vi "HW_GEN - Write Module Channel Configurations(bin).vi"(8 "error in":errorcluster caption="错误输入", 10 "ModuCfg":T1[](array[typedef]), 11 "Path":path) -> (0 "error out":errorcluster caption="错误输出")   [LabVIEW 2016]
uses:
  Ctrls/HardWare _ Module Configuration.ctl
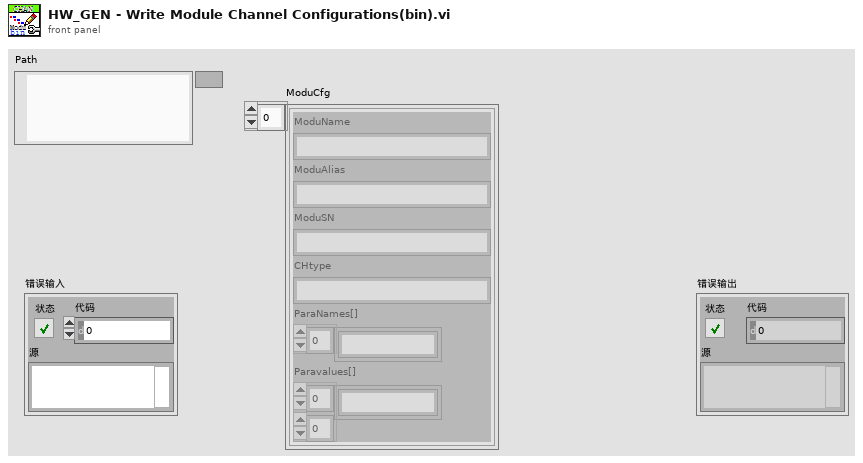
[diagram p1: front panel]
types:
  T1 = typedef "HardWare _ Module Configuration.ctl" = cluster{"ModuName":string, "ModuAlias":string, "ModuSN":string, "CHtype":string, "ParaNames[]":string[], "Paravalues[]":string[][]}
  T2 = enum16{"open", "replace", "create", "open or create", "replace or create", "replace or create with confirmation"}
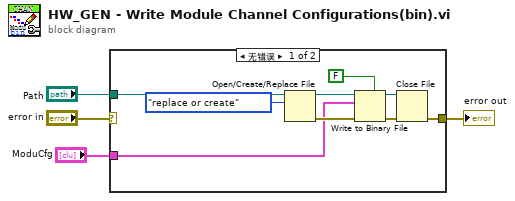
[diagram p0: block diagram]
diagram:
  n1 = case shown="无错误" "error in" {
    selector: "error in" -> [_ w14]
    tunnel: [w11 w14] -> w2
    tunnel: "Path" -> [w12 _]
    tunnel: "ModuCfg" -> [w8 _]
    frame No Error {
      n2 = Open/Create/Replace File(file path (use dialog)=w12, operation (0:open)=T2."replace or create" ("操作(0:open)")) -> (refnum out=w9:refnum<file>, error out=w10:errorcluster)  [unwired: 4 in, 1 out]
      n3 = Write to Binary File(file (use dialog)=w9, data=w8, error in=w10, 5:FALSE ("prepend array or string size? (T)")) -> (refnum out=w5:refnum<file>, error out=w6:errorcluster)  [unwired: 2 in, 1 out]
      n4 = Close File(refnum=w5, error in=w6) -> (error out=w11:errorcluster)  [unwired: 1 out]
    }
    frame Error {
    }
  }
  "error out" <- w2
